vi "ModelParameterValueGet.vi"(9 "Target":string, 10 "Parameter":string, 11 "ModelManager in":T1) -> (0 "error out":errorcluster, 1 "Target out":string, 2 "Parameter name out":string, 3 "Value":dbl)   [LabVIEW 2015, in "MiscHelperVIs.lvlib"]
uses:
  MiscHelperVIs.lvlib
  <vilib>/NI Veristand/Execution/ModelManager/ModelManagerAPI.ctl
  NationalInstruments.VeriStand.ClientAPI
  <vilib>/NI Veristand/Execution/ModelManager/NI VeriStand - Get Single Parameter Value.vi
  <vilib>/NI Veristand/Execution/ModelManager/NI_VS ModelManager ExecutionAPI.lvlib
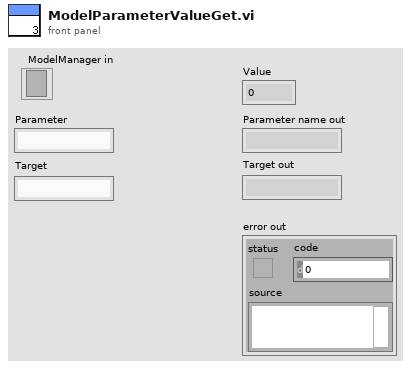
[diagram p1: front panel]
types:
  T1 = typedef "NI_VS ModelManager ExecutionAPI.lvlib/ModelManagerAPI.ctl" = refnum<k24>
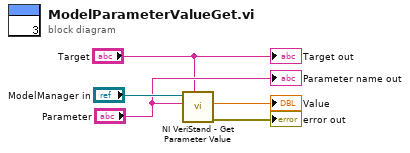
[diagram p0: block diagram]
diagram:
  n1 = call-poly <vilib>:"NI VeriStand - Get Parameter Value.vi"("Target"="Target", "Parameter"="Parameter", "ModelManager in"="ModelManager in") -> ("error out"=→"error out":errorcluster, "Value"=→"Value":dbl)  [unwired: 6 in, 1 out]
  "Parameter name out" <- "Parameter"
  "Target out" <- "Target"
